vi "VI Name.vi"(11 "VI":refnum<vi>) -> (3 "VI Name":string)   [LabVIEW 2017, in "DSF Core.lvlib"]
uses:
  DSF Core.lvlib
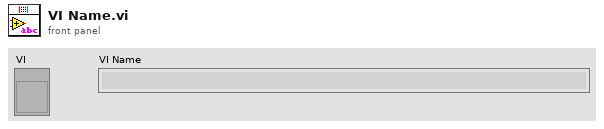
[diagram p1: front panel]
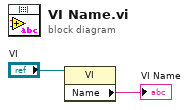
[diagram p0: block diagram]
diagram:
  n1 = property class="VI"(reference="VI") -> ("Name"=→"VI Name":string)  [unwired: 1 in, 2 out]
